vi "Read.vi"(8 "error in (no error)":errorcluster, 11 "ConvertTo in":refnum<class "ConvertTo_String.lvclass">) -> (0 "error out":errorcluster, 2 "Value":string, 3 "ConvertTo out":refnum<class "ConvertTo_String.lvclass">)   [LabVIEW 2021, in "ConvertTo_String.lvclass"]
uses:
  ConvertTo_String.lvclass
  ConvertTo_String.lvclass/ConvertTo_String.ctl
  Properties/Read Value.vi
  Properties/Write Value.vi
  Abs_Types/Value/Abs_Value.lvclass
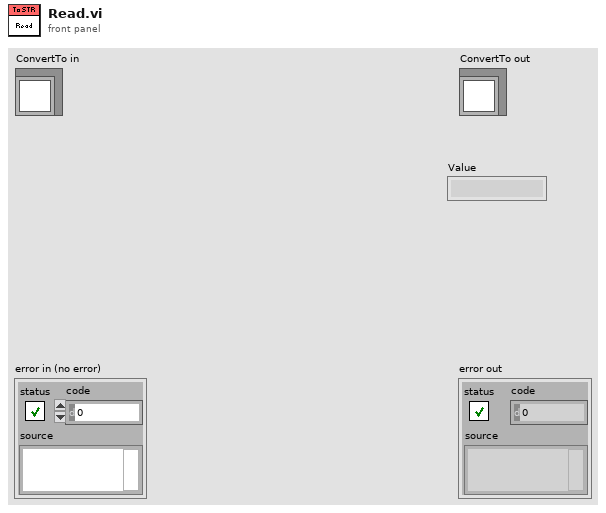
[diagram p1: front panel]
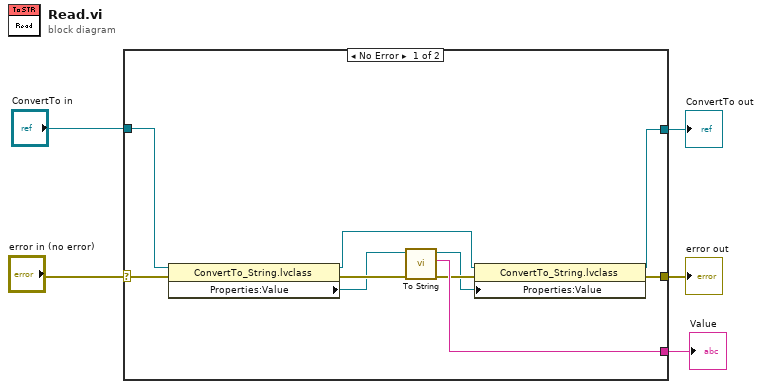
[diagram p0: block diagram]
diagram:
  n1 = case shown="No Error" "error in (no error)" {
    selector: "error in (no error)" -> [w15 w16]
    tunnel: "ConvertTo in" -> [w14 w17]
    tunnel: [w11 _] -> w3
    tunnel: [w7 w16] -> w2
    tunnel: [w6 w17] -> w1
    frame No Error {
      n2 = property class="ConvertTo_String.lvclass"(reference=w14, error in=w15) -> (reference out=w10:refnum<class "ConvertTo_String.lvclass">, error out=w13:errorcluster, "Properties:Value"=w12:refnum<class "Abs_Value.lvclass">)
      n3 = call-dynamic "To String.vi"("error in (no error)"=w13, "Types in"=w12) -> ("error out"=w9:errorcluster, "String"=w11:string, "Types out"=w8:refnum<class "Abs_Value.lvclass">)  [unwired: 7 in]
      n4 = property class="ConvertTo_String.lvclass"(reference=w10, error in=w9, "Properties:Value"=w8) -> (reference out=w6:refnum<class "ConvertTo_String.lvclass">, error out=w7:errorcluster)
    }
    frame Error {
    }
  }
  "error out" <- w2
  "ConvertTo out" <- w1
  "Value" <- w3
